vi "Convert Angle to Pulse Width.vi"(10 "ccw angle offset (rad)":fxp<+/-,32,4>, 11 "ccw angle (rad)":fxp<+/-,32,4>) -> (3 "pulse width (uSec)":u32)   [LabVIEW 2013, in "NI_Robotics_Hitec HS400 Series (FPGA).lvlib"]
doc: "Converts the angle in rad to the pulse width in us."
uses:
  NI_Robotics_Hitec HS400 Series (FPGA).lvlib
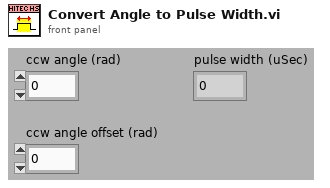
[diagram p1: front panel]
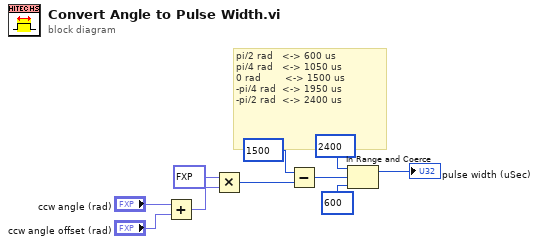
[diagram p0: block diagram]
diagram:
  # "pi/2 rad   <-> 600 us\npi/4 rad   <-> 1050 us\n0 rad        <-> 1500 us\n-pi/4 rad  <-> 1950 us\n-pi/2 rad  <-> 2400 us"
  n1 = Add(x="ccw angle (rad)", y="ccw angle offset (rad)") -> (x+y=w7:fxp<+/-,33,5>)
  n2 = Multiply(x=fxp<+,10,10> 573.0 ("angle (rad)"), y=w7) -> (x*y=w2:i32)
  n3 = Subtract(x=1500 ("y"), y=w2) -> (x-y=w10:i32)
  n4 = In Range and Coerce(upper limit=2400, x=w10, lower limit=600) -> (coerced(x)=→"pulse width (uSec)":i32)  [unwired: 1 out]
